vi "ATS_Get_Specs.vi"(8 "InputControl":T5 {"Range" items=["20mV", "40mV", "50mV", "80mV", "100mV", "200mV", "400mV", "500mV", "800mV", "1 V", "1.25 V", "2 V", "4 V", "5 V", "8 V", "10 V", "16 V", "20 V", "40 V", "HiFi"]}, 10 "Clock_Input":T1 {"ClckEdge" items=["Rising", "Falling"]; "ClckRate" items=["1 kS/s", "2 kS/s", "5 kS/s", "10 kS/s", "20 kS/s", "50 kS/s", "100 kS/s", "200 kS/s", "500 kS/s", "1 MS/s", "2 MS/s", "5 MS/s", "10 MS/s", "20 MS/s", "25 MS/s", "50 MS/s", "100 MS/s", "125 MS/s", "200 MS/s", "250 MS/s", "500 MS/s", "1 GS/s"]}, 11 "ID":i32) -> (1 "Range_Out":cluster{"Text":string, "Range":u32}, 2 "Rate_Out":cluster{"Text":string, "Rate":u32}, 3 "Card_Spec":T10, 6 "OutputControl":T5 {"Range" items=["20mV", "40mV", "50mV", "80mV", "100mV", "200mV", "400mV", "500mV", "800mV", "1 V", "1.25 V", "2 V", "4 V", "5 V", "8 V", "10 V", "16 V", "20 V", "40 V", "HiFi"]}, 7 "Clock_Output":T1 {"ClckEdge" items=["Rising", "Falling"]; "ClckRate" items=["1 kS/s", "2 kS/s", "5 kS/s", "10 kS/s", "20 kS/s", "50 kS/s", "100 kS/s", "200 kS/s", "500 kS/s", "1 MS/s", "2 MS/s", "5 MS/s", "10 MS/s", "20 MS/s", "25 MS/s", "50 MS/s", "100 MS/s", "125 MS/s", "200 MS/s", "250 MS/s", "500 MS/s", "1 GS/s"]})   [LabVIEW 2010]
doc: "_____AlazarTech, Scope_____\n\nGet the Specification of the board ID.\n\nInput:\n\"ID\" = Board to get the specification\n\"Rate_In\" = select the sampling rate (value limited by the max of the Card_Spec)\n can be Index or Sampling Rate in Hz.\n\"Range_In\" = select the input range (value limited by the max of the Card_Spec\n can be Index or Voltage value in mV.\n\nOutput\n\"Card_Spec\" = specification of the board.\n \"Name\" = string of the ATS board identification\n \"Rate\" = list of available Sampling Rate in a string array format\n \"Range\" = list of available Input range in a string array format\n\"Rate_Out\" = sampling rate selected by Rate_In in text and value format\n\"Range_Out\" = input range selected by Range_In in text and value format"
uses:
  ATS_ctl/ATS_Card_Spec.ctl
  ATS_ctl/InputCtrl.ctl
  ATS_ctl/Coupling.ctl
  ATS_ctl/Range.ctl
  ATS_ctl/Impedance.ctl
  ATS_ctl/Bandwidth.ctl
  ATS_ctl/Clock.ctl
  ATS_ctl/ClockSource.ctl
  ATS_ctl/ClockRate.ctl
  ATS_ctl/ClockEdge.ctl
  ATS_ctl/ATS_Spec_Selector.ctl
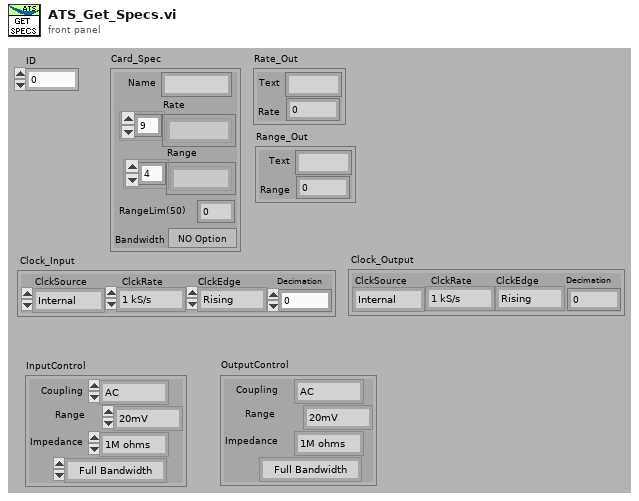
[diagram p1: front panel]
types:
  T1 = typedef "Clock.ctl" = cluster{"ClckSource":T2, "ClckRate":T3, "ClckEdge":T4, "Decimation":u32}
  T2 = typedef "ClockSource.ctl" = enum16{"Internal", "External", "Medium Ext.", "Slow Ext.", "Ext. AC", "Ext. DC", "Ext. (PLL)"}
  T3 = typedef "ClockRate.ctl" = u32
  T4 = typedef "ClockEdge.ctl" = u16
  T5 = typedef "InputCtrl.ctl" = cluster{"Coupling":T6, "Range":T7, "Impedance":T8, "Bandwidth":T9}
  T6 = typedef "Coupling.ctl" = enum16{"AC", "DC"}
  T7 = typedef "Range.ctl" = u32
  T8 = typedef "Impedance.ctl" = enum16{"1M ohms", "50 ohms"}
  T9 = typedef "Bandwidth.ctl" = enum16{"Full Bandwidth", "Reduce Bandwidth"}
  T10 = typedef "ATS_Card_Spec.ctl" = cluster{"Name":string, "Rate":string[], "Range":string[], "RangeLim(50)":u32, "Bandwidth":bool}
  T11 = typedef "ATS_Spec_Selector.ctl" = enum16{"None", "ClckSource", "ClckEdge", "ClckRate", "InputRange", "InputCoupling", "Impedance", "Bandwidth", "AsyncDMA", "Memory", "ExtTrigCoupling", "ExtTrigRange", "AUX_IO_Trig", "AUX_IO_Slope", "Trigger_Source"}
  T12 = typedef "ATS_Global_Specs_Ctrl.ctl" = cluster{"ClckSource":cluster{"Internal":bool, "External":bool, "Medium Ext.":bool, "Slow Ext.":bool, "Ext. AC":bool, "Ext. DC":bool, "Ext. (PLL)":bool}, "ClckRate":cluster{"1 kS/s":bool, "2 kS/s":bool, "5 kS/s":bool, "10 kS/s":bool, "20 kS/s":bool, "50 kS/s":bool, "100 kS/s":bool, "200 kS/s":bool, "500 kS/s":bool, "1 MS/s":bool, "2 MS/s":bool, "5 MS/s":bool, "10 MS/s":bool, "20 MS/s":bool, "25 MS/s":bool, "50 MS/s":bool, "100 MS/s":bool, "125 MS/s":bool, "160 MS/s":bool, "180 MS/s":bool, "200 MS/s":bool, "250 MS/s":bool, "500 MS/s":bool, "1 GS/s":bool}, "ClckEdge":cluster{"Rising":bool, "Falling":bool}, "InputCoupling":cluster{"AC":bool, "DC":bool}, "InputRange":cluster{"20mV":bool, "40mV":bool, "50mV":bool, "80mV":bool, "100mV":bool, "200mV":bool, "400mV":bool, "500mV":bool, "800mV":bool, "1 V":bool, "2 V":bool, "4 V":bool, "5 V":bool, "8 V":bool, "10 V":bool, "16 V":bool, "20 V":bool, "40 V":bool, "HiFi":bool, "1.25 V":bool}, "Impedance":cluster{"1M ohms":bool, "50 ohms":bool, "300 ohms":bool}, "Bandwidth":cluster{"Full":bool, "Reduce":bool}, "RangeLim(50)":string, "AsyncDMA":cluster{"OnBoard":bool, "FPGA":bool}, "Memory":cluster{"VerifMem":bool, "HighMem":bool, "Combine":bool, "HighRecord":bool}, "ExtTrigCoupling":cluster{"AC":bool, "DC":bool}, "ExtTrigRange":cluster{"1 V":bool, "5 V":bool, "\nTTL":bool}, "AUX_IO_Trig":cluster{"Trig_Out":bool, "Trig_In":bool}, "AUX_IO_Slope":cluster{"Rising":bool, "Falling":bool}, "MaxPretrig":cluster{"MEM":u32, "FIFO":u32}, "AUX_I/O_Trig":cluster{"OUT_Trigger":bool, "OUT_PACER":bool, "OUT_BUSY":bool, "OUT_CLOCK":bool, "OUT_RESERVED":bool, "OUT_CAPTURE_ALMOST_DONE":bool, "OUT_AUXILIARY":bool, "OUT_SERIAL_DATA":bool, "IN_TRIGGER_ENABLE":bool, "IN_DIGITAL_TRIGGER":bool, "IN_GATE":bool, "IN_CAPTURE_ON_DEMAND":bool, "IN_RESET_TIMESTAMP":bool, "IN_SLOW_EXTERNAL_CLOCK":bool, "INPUT_AUXILIARY":bool, "INPUT_SERIAL_DATA":bool}, "ChannelsPerBoard":u8}
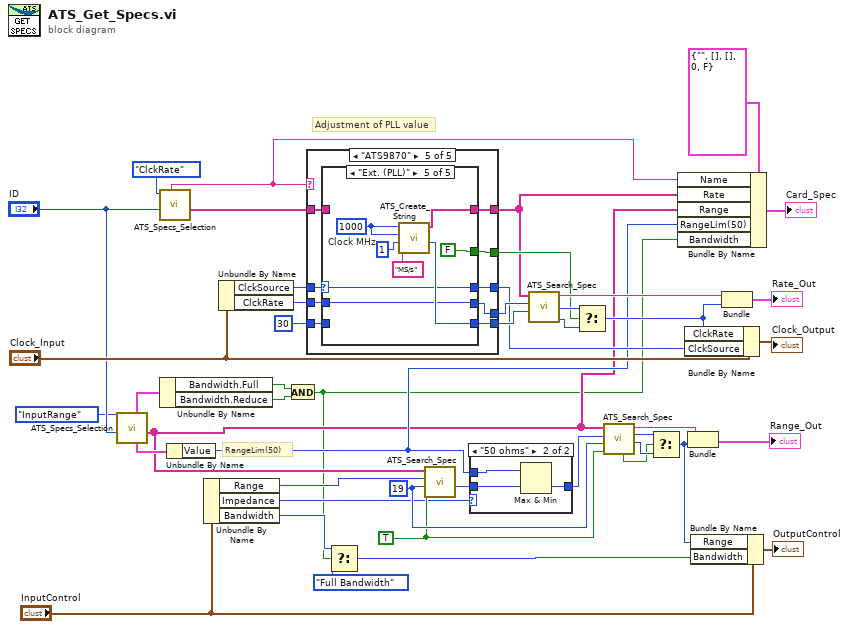
[diagram p0: block diagram]
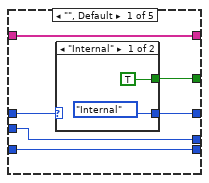
[diagram p2: hidden frame]
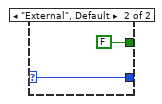
[diagram p3: hidden frame]
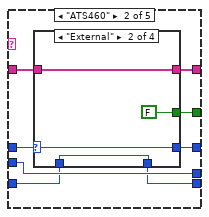
[diagram p4: hidden frame]
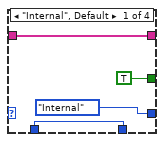
[diagram p5: hidden frame]
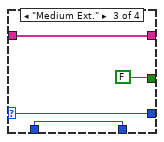
[diagram p6: hidden frame]
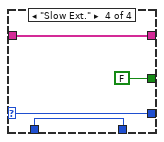
[diagram p7: hidden frame]
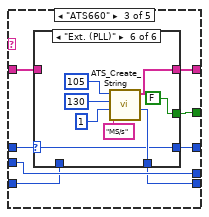
[diagram p8: hidden frame]
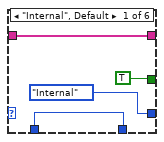
[diagram p9: hidden frame]
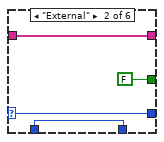
[diagram p10: hidden frame]
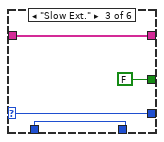
[diagram p11: hidden frame]
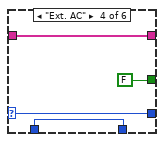
[diagram p12: hidden frame]
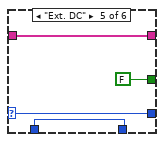
[diagram p13: hidden frame]
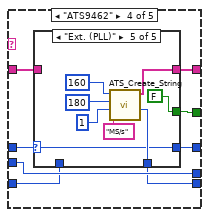
[diagram p14: hidden frame]
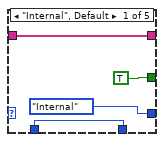
[diagram p15: hidden frame]
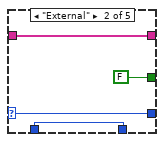
[diagram p16: hidden frame]
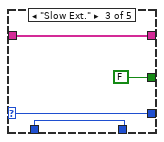
[diagram p17: hidden frame]
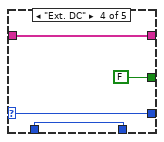
[diagram p18: hidden frame]
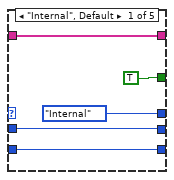
[diagram p19: hidden frame]
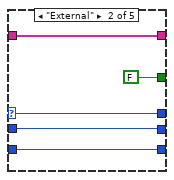
[diagram p20: hidden frame]
diagram:
  w40 = TRUE ("Rate / Range")
  w41 = u32 19 ("Treshold (30)")
  # "RangeLim(50)"
  # "Adjustment of PLL value"
  n1 = call "ATS_Specs_Selection.vi"("ID"="ID", "ATS_Spec_Selector"=ATS_Spec_Selector."InputRange") -> ("Possible_Item"=w9:string[], "Other"=w15:cluster{"ValueName":string, "Value":u32}, "Specifications"=w6:T12)  [unwired: 3 in, 4 out]
  n2 = call "ATS_Specs_Selection.vi"("ID"="ID", "ATS_Spec_Selector"=ATS_Spec_Selector."ClckRate") -> ("Possible_Item"=w8:string[], "Device_Name"=w3:string)  [unwired: 3 in, 5 out]
  n3 = Unbundle By Name(w6) -> ("Bandwidth.Full"=w5:bool, "Bandwidth.Reduce"=w4:bool)
  n4 = Unbundle By Name(w15) -> ("Value"=w10:u32)
  n5 = Unbundle By Name("InputControl") -> ("Range"=w35:T7, "Impedance"=w34:T8, "Bandwidth"=w33:T9)
  n6 = Unbundle By Name("Clock_Input") -> ("ClckSource"=w22:T2, "ClckRate"=w29:T3)
  n7 = And(x=w5, y=w4) -> (x .and. y?=w2:bool)
  n8 = case shown="\"ATS9870\"" w3 {
    tunnel: w29 -> [w51 w61 w85 w121 w150]
    tunnel: w22 -> [w49 w64 w88 w124 w157]
    tunnel: u32 30 ("Treshold (30)") -> [w50 w59 w83 w119 w153]
    tunnel: w8 -> [w52 w63 w87 w123 w156]
    tunnel: [w52 w62 w86 w122 w155] -> w7
    tunnel: [w50 w60 w84 w120 w154] -> w24
    tunnel: [w51 w61 w85 w121 w149] -> w23
    tunnel: [w48 w58 w82 w118 w152] -> w21
    tunnel: [w47 w57 w81 w117 w151] -> w16
    frame "", Default {
      n9 = case shown="\"Internal\"" w49 {
        selector: w49 -> [_ w56]
        tunnel: [ClockSource."Internal" ("ClckSource") w56] -> w48
        tunnel: [TRUE ("s") FALSE ("s")] -> w47
        frame "Internal" {
        }
        frame "External", Default {
        }
      }
    }
    frame "ATS460" {
      n10 = case shown="\"External\"" w64 {
        selector: w64 -> [_ w70 w74 w78]
        tunnel: w63 -> [w68 w72 w76 w80]
        tunnel: [w68 w72 w76 w80] -> w62
        tunnel: [w67 w71 w75 w79] -> w60
        tunnel: w59 -> [w67 w71 w75 w79]
        tunnel: [ClockSource."Internal" ("ClckSource") w70 w74 w78] -> w58
        tunnel: [TRUE ("s") FALSE ("s") FALSE ("s") FALSE ("s")] -> w57
        frame "Internal", Default {
        }
        frame "External" {
        }
        frame "Medium Ext." {
        }
        frame "Slow Ext." {
        }
      }
    }
    frame "ATS660" {
      n11 = case shown="\"Ext. (PLL)\"" w88 {
        selector: w88 -> [_ w94 w98 w102 w106 w111]
        tunnel: w87 -> [w92 w96 w100 w104 w108 _]
        tunnel: [w92 w96 w100 w104 w108 w109] -> w86
        tunnel: [w91 w95 w99 w103 w107 w112] -> w84
        tunnel: w83 -> [w91 w95 w99 w103 w107 _]
        tunnel: [ClockSource."Internal" ("ClckSource") w94 w98 w102 w106 w111] -> w82
        tunnel: [TRUE ("s") FALSE ("s") FALSE ("s") FALSE ("s") FALSE ("s") FALSE ("s")] -> w81
        frame "Internal", Default {
        }
        frame "External" {
        }
        frame "Slow Ext." {
        }
        frame "Ext. AC" {
        }
        frame "Ext. DC" {
        }
        frame "Ext. (PLL)" {
          n12 = call "ATS_Create_String.vi"("Scale"="MS/s", "Step"=1, "End"=130, "Start"=105) -> ("Count"=w112:u32, "Range_Out"=w109:string[])  [unwired: 6 in]
        }
      }
    }
    frame "ATS9462" {
      n13 = case shown="\"Ext. (PLL)\"" w124 {
        selector: w124 -> [_ w130 w134 w138 w144]
        tunnel: w123 -> [w128 w132 w136 w140 _]
        tunnel: [w128 w132 w136 w140 w145] -> w122
        tunnel: [w127 w131 w135 w139 w147] -> w120
        tunnel: w119 -> [w127 w131 w135 w139 _]
        tunnel: [ClockSource."Internal" ("ClckSource") w130 w134 w138 w144] -> w118
        tunnel: [TRUE ("s") FALSE ("s") FALSE ("s") FALSE ("s") FALSE ("s")] -> w117
        frame "Internal", Default {
        }
        frame "External" {
        }
        frame "Slow Ext." {
        }
        frame "Ext. DC" {
        }
        frame "Ext. (PLL)" {
          n14 = call "ATS_Create_String.vi"("Scale"="MS/s", "Step"=1, "End"=180, "Start"=160) -> ("Count"=w147:u32, "Range_Out"=w145:string[])  [unwired: 6 in]
        }
      }
    }
    frame "ATS9870" {
      n15 = case shown="\"Ext. (PLL)\"" w157 {
        selector: w157 -> [_ w165 w170 w175 w183]
        tunnel: w156 -> [w162 w167 w172 w177 _]
        tunnel: [w162 w167 w172 w177 w181] -> w155
        tunnel: [w161 w166 w171 w176 w184] -> w154
        tunnel: w153 -> [w161 w166 w171 w176 _]
        tunnel: [ClockSource."Internal" ("ClckSource") w165 w170 w175 w183] -> w152
        tunnel: [TRUE ("s") FALSE ("s") FALSE ("s") FALSE ("s") FALSE ("s")] -> w151
        tunnel: w150 -> [w158 w163 w168 w173 w178]
        tunnel: [w158 w163 w168 w173 w178] -> w149
        frame "Internal", Default {
        }
        frame "External" {
        }
        frame "Ext. AC" {
        }
        frame "Ext. DC" {
        }
        frame "Ext. (PLL)" {
          w179 = 1000  # Clock MHz
          n16 = call "ATS_Create_String.vi"("Scale"="MS/s", "Step"=1, "End"=w179, "Start"=w179) -> ("Count"=w184:u32, "Range_Out"=w181:string[])  [unwired: 6 in]
        }
      }
    }
  }
  n17 = Select(t=w33, s=w2, f=Bandwidth."Full Bandwidth" ("Bandwidth")) -> (s? t:f=w31:T9)
  n18 = call "ATS_Search_Spec.vi"("Rate / Range"=w40, "Treshold (30)"=w41, "Value In"=w35, "StringArray"=w9) -> ("Index"=w43:u32)  [unwired: 3 in, 4 out]
  n19 = case shown="\"50 ohms\"" w34 {
    tunnel: w43 -> [w186 w189]
    tunnel: w10 -> [_ w188]
    tunnel: [w186 w187] -> w42
    frame "1M ohms", Default {
    }
    frame "50 ohms" {
      n20 = Max & Min(x=w188, y=w189) -> (min(x,y)=w187:u32)  [unwired: 1 out]
    }
  }
  n21 = call "ATS_Search_Spec.vi"("Treshold (30)"=w24, "Value In"=w23, "StringArray"=w7) -> ("Result"=w19:u32, "Index"=w18:u32, "String"=w25:string)  [unwired: 4 in, 2 out]
  n22 = Select(t=w18, s=w16, f=w19) -> (s? t:f=w17:u32)
  n23 = call "ATS_Search_Spec.vi"("Rate / Range"=w40, "Treshold (30)"=w41, "Value In"=w42, "StringArray"=w9) -> ("Index"=w38:u32, "Out_Value"=w39:u32, "String"=w44:string, ">Treshold"=w20:bool)  [unwired: 3 in, 1 out]
  n24 = Select(t=w39, s=w20, f=w38) -> (s? t:f=w30:u32)
  n25 = Bundle By Name(cluster=T10 {"Name"="", "Rate"=[], "Range"=[], "RangeLim(50)"=0, "Bandwidth"=FALSE} ("Card_Spec"), "Name"=w3, "Rate"=w7, "Range"=w9, "RangeLim(50)"=w10, "Bandwidth"=w2) -> (→"Card_Spec":T10)
  n26 = Bundle By Name(cluster="Clock_Input", "ClckRate"=w17, "ClckSource"=w21) -> (→"Clock_Output":T1)
  n27 = Bundle("String"=w44, "Index"=w30) -> (→"Range_Out":cluster{"String":string, "Index":u32})  [unwired: 1 in]
  n28 = Bundle By Name(cluster="InputControl", "Range"=w30, "Bandwidth"=w31) -> (→"OutputControl":T5)
  n29 = Bundle("String"=w25, "Result"=w17) -> (→"Rate_Out":cluster{"String":string, "Result":u32})  [unwired: 1 in]
